vi "Visualise Lines.vi"(11 "Lines":T1[](array[typedef])) -> (3 "XY Graph":cluster{dbl[], dbl[]}[](graph))   [LabVIEW 2017]
uses:
  Vector Library/Line.ctl
  Vector Library/Vector.ctl
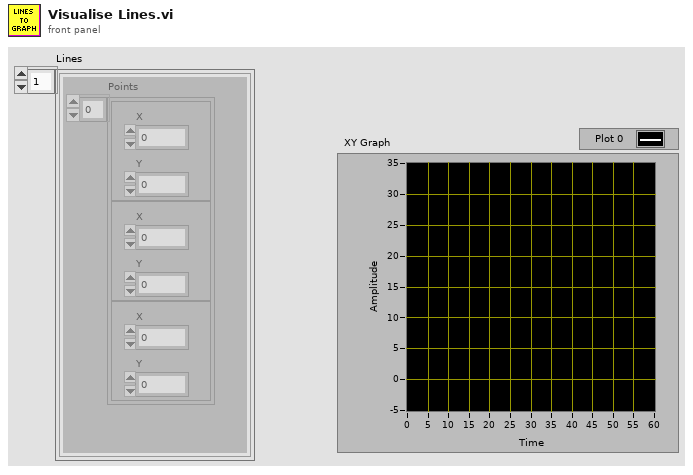
[diagram p1: front panel]
types:
  T1 = typedef "Line.ctl" = cluster{"Points":T2[]}
  T2 = typedef "Vector.ctl" = cluster{"X":dbl, "Y":dbl}
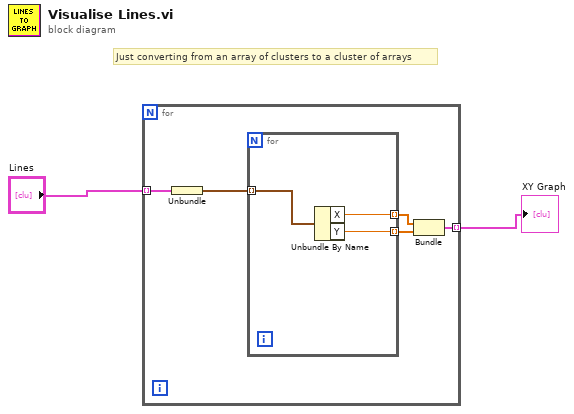
[diagram p0: block diagram]
diagram:
  # "Just converting from an array of clusters to a cluster of arrays"
  n1 = for {
    tunnel: "Lines" -> [w7] mode=indexing
    tunnel: [w3] -> w1 mode=indexing
    n2 = Unbundle(w7) -> ("Points"=w6:T2[])
    n3 = for {
      tunnel: w6 -> [w10] mode=indexing
      tunnel: [w9] -> w5 mode=indexing
      tunnel: [w8] -> w4 mode=indexing
      n4 = Unbundle By Name(w10) -> ("X"=w9:dbl, "Y"=w8:dbl)
    }
    n5 = Bundle(w5, w4) -> (w3:cluster{dbl[], dbl[]})  [unwired: 1 in]
  }
  "XY Graph" <- w1
